vi "test Set Parity.vi"(8 "error in (no error)":errorcluster, 11 "TestCase in":refnum<class "Parity.lvclass">) -> (0 "error out":errorcluster, 3 "TestCase out":refnum<class "Parity.lvclass">)   [LabVIEW 2027, in "Parity.lvclass"]
uses:
  Parity.lvclass
  Source/Parity.ctl
  ca462cc8-d8fc-406a-9a43-00fa4182e3f2.vi
  96d02928-22ca-436d-b71e-df342981c4d4.vi
  3e59ff5b-2dac-40d5-8915-f6dafffb65a4.vi
  418561d5-1643-4c38-8e71-5b42483485ba.vi
  69d58664-bd3b-4127-acca-004e0ada79b4.vi
  1f118f69-e861-4846-b08f-373b0f5f84dc.vi
  08562fc9-d800-4538-b7a4-3d12455cbaf0.vi
  e69cf9e1-9200-45b3-811d-d0e4d2f0e09e.vi
  b79821fd-afdc-4fd3-a910-5010e2989e8e.vi
  004fd942-893e-4146-9c65-8ea3c19e933b.vi
  977484d6-27d9-45ec-8210-9f77f2740aaf.vi
  C:/Program Files/National Instruments/LabVIEW 2027/vi.lib/addons/_JKI Toolkits/VI Tester/TestCase.llb/TestCase.lvclass
  <vilib>/addons/_JKI Toolkits/VI Tester/TestCase.llb/TestCase.lvclass
  Source/Encoding and Decoding.lvlib
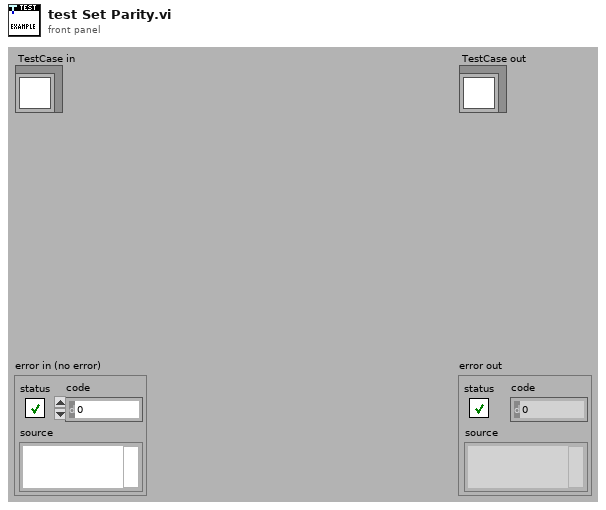
[diagram p1: front panel]
types:
  T1 = typedef "Encoding and Decoding.lvlib/Parity.ctl" = enum16{"Even", "Odd"}
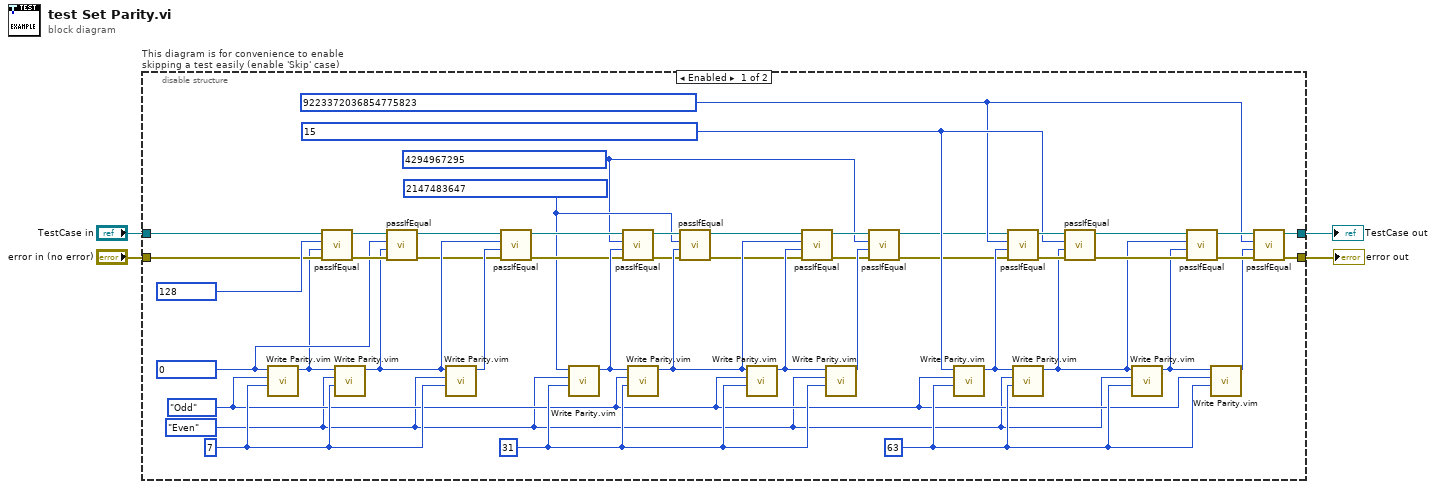
[diagram p0: block diagram]
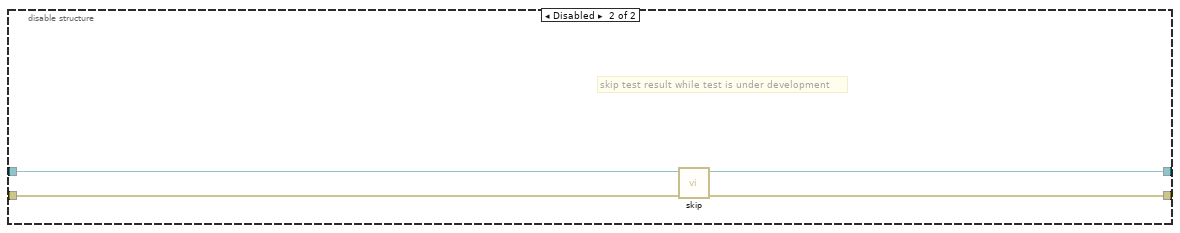
[diagram p2: hidden frame]
diagram:
  n1 = disable-structure "This diagram is for convenience to enable skipping a test easily (enable 'Skip' case)" shown="Enabled" {
    disable-tunnel: "TestCase in" -> [w50 w54]
    disable-tunnel: [w33 w52] -> w1
    disable-tunnel: [w28 w53] -> w3
    disable-tunnel: "error in (no error)" -> [w46 w51]
    frame Enabled {
      w10 = u32 2147483647 ("word in")
      w9 = u32 4294967295 ("word in")
      w20 = 31 ("parity index")
      w27 = u64 15 ("word in")
      w24 = u64 9223372036854775823 ("word in")
      w30 = 63 ("parity index")
      w5 = Parity."Even" ("parity")
      w43 = 7 ("parity index")
      w6 = Parity."Odd" ("parity")
      w45 = u8 0 ("word in")
      n2 = call "Write Parity.vim"("parity index"=w43, "parity"=w6, "word in"=w45) -> ("word out"=w44:u8)  [unwired: 8 in]
      n3 = call-dynamic "passIfEqual.vi"("error in (no error)"=w46, "y"=w44, "x"=u8 128 ("word in"), "TestCase in"=w50) -> ("error out"=w47:errorcluster, "TestCase out"=w48:refnum<class "Parity.lvclass">)  [unwired: 6 in]
      n4 = call "Write Parity.vim"("parity index"=w43, "parity"=w5, "word in"=w44) -> ("word out"=w41:u8)  [unwired: 8 in]
      n5 = call-dynamic "passIfEqual.vi"("error in (no error)"=w47, "y"=w41, "x"=w45, "TestCase in"=w48) -> ("error out"=w39:errorcluster, "TestCase out"=w40:refnum<class "Parity.lvclass">)  [unwired: 6 in]
      n6 = call "Write Parity.vim"("parity index"=w43, "parity"=w5, "word in"=w41) -> ("word out"=w42:u8)  [unwired: 8 in]
      n7 = call-dynamic "passIfEqual.vi"("error in (no error)"=w39, "y"=w42, "x"=w41, "TestCase in"=w40) -> ("error out"=w11:errorcluster, "TestCase out"=w12:refnum<class "Parity.lvclass">)  [unwired: 6 in]
      n8 = call "Write Parity.vim"("parity index"=w20, "parity"=w5, "word in"=w10) -> ("word out"=w22:u32)  [unwired: 8 in]
      n9 = call-dynamic "passIfEqual.vi"("error in (no error)"=w11, "y"=w22, "x"=w9, "TestCase in"=w12) -> ("error out"=w15:errorcluster, "TestCase out"=w16:refnum<class "Parity.lvclass">)  [unwired: 6 in]
      n10 = call "Write Parity.vim"("parity index"=w20, "parity"=w6, "word in"=w22) -> ("word out"=w23:u32)  [unwired: 8 in]
      n11 = call-dynamic "passIfEqual.vi"("error in (no error)"=w15, "y"=w23, "x"=w10, "TestCase in"=w16) -> ("error out"=w13:errorcluster, "TestCase out"=w14:refnum<class "Parity.lvclass">)  [unwired: 6 in]
      n12 = call "Write Parity.vim"("parity index"=w20, "parity"=w6, "word in"=w23) -> ("word out"=w17:u32)  [unwired: 8 in]
      n13 = call-dynamic "passIfEqual.vi"("error in (no error)"=w13, "y"=w17, "x"=w23, "TestCase in"=w14) -> ("error out"=w19:errorcluster, "TestCase out"=w18:refnum<class "Parity.lvclass">)  [unwired: 6 in]
      n14 = call "Write Parity.vim"("parity index"=w20, "parity"=w5, "word in"=w17) -> ("word out"=w21:u32)  [unwired: 8 in]
      n15 = call-dynamic "passIfEqual.vi"("error in (no error)"=w19, "y"=w21, "x"=w9, "TestCase in"=w18) -> ("error out"=w7:errorcluster, "TestCase out"=w8:refnum<class "Parity.lvclass">)  [unwired: 6 in]
      n16 = call "Write Parity.vim"("parity index"=w30, "parity"=w6, "word in"=w27) -> ("word out"=w26:u64)  [unwired: 8 in]
      n17 = call-dynamic "passIfEqual.vi"("error in (no error)"=w7, "y"=w26, "x"=w24, "TestCase in"=w8) -> ("error out"=w36:errorcluster, "TestCase out"=w35:refnum<class "Parity.lvclass">)  [unwired: 6 in]
      n18 = call "Write Parity.vim"("parity index"=w30, "parity"=w5, "word in"=w26) -> ("word out"=w25:u64)  [unwired: 8 in]
      n19 = call-dynamic "passIfEqual.vi"("error in (no error)"=w36, "y"=w25, "x"=w27, "TestCase in"=w35) -> ("error out"=w38:errorcluster, "TestCase out"=w37:refnum<class "Parity.lvclass">)  [unwired: 6 in]
      n20 = call "Write Parity.vim"("parity index"=w30, "parity"=w5, "word in"=w25) -> ("word out"=w34:u64)  [unwired: 8 in]
      n21 = call-dynamic "passIfEqual.vi"("error in (no error)"=w38, "y"=w34, "x"=w25, "TestCase in"=w37) -> ("error out"=w31:errorcluster, "TestCase out"=w32:refnum<class "Parity.lvclass">)  [unwired: 6 in]
      n22 = call "Write Parity.vim"("parity index"=w30, "parity"=w6, "word in"=w34) -> ("word out"=w29:u64)  [unwired: 8 in]
      n23 = call-dynamic "passIfEqual.vi"("error in (no error)"=w31, "y"=w29, "x"=w24, "TestCase in"=w32) -> ("error out"=w28:errorcluster, "TestCase out"=w33:refnum<class "Parity.lvclass">)  [unwired: 6 in]
    }
    frame Disabled {
      # "skip test result while test is under development"
      n24 = call <vilib>:"skip.vi"("error in (no error)"=w51, "TestCase in"=w54) -> ("error out"=w53:errorcluster, "TestCase out"=w52:refnum<class "Parity.lvclass">)  [unwired: 8 in]
    }
  }
  "error out" <- w3
  "TestCase out" <- w1
